vi "Drive GetSensors.vi"(1 "Drive Global Data In":T1) -> (0 "Drive Global Data Out":T1)   [LabVIEW 2013]
panel:
  in  "wheel diameteres":dbl
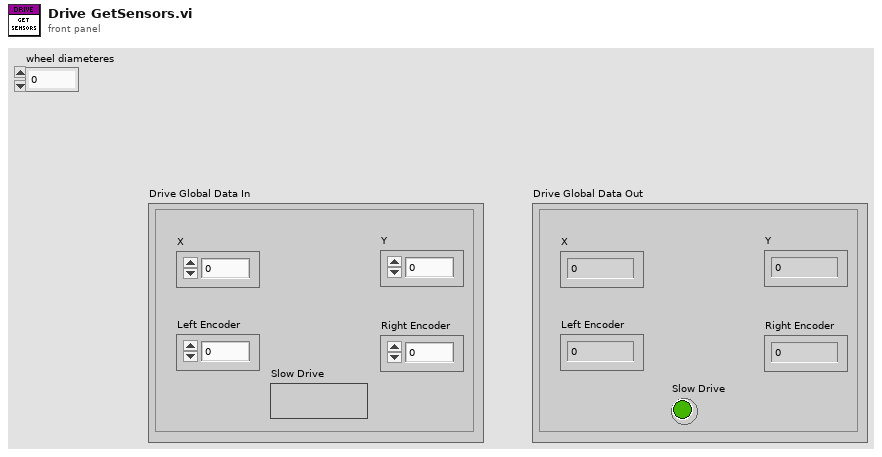
[diagram p1: front panel]
types:
  T1 = cluster{"Y":dbl, "X":dbl, "Left Encoder":dbl, "Right Encoder":dbl, "Slow Drive":bool}
  T2 = typedef "WPI_EncoderDevRef.ctl" = cluster{"DevStatus":errorcluster, "EncoderIndex":T3, "CounterIndex":T4, "DistancePerCount":dbl, "Decoding Type":T5}
  T3 = typedef "FPGA_EncoderIdx.ctl" = enum8{"Enc 0", "Enc 1", "Enc 2", "Enc 3", "Invalid"}
  T4 = typedef "FPGA_CounterCtrSystemIndex.ctl" = enum8{"Ctr 0", "Ctr 1", "Ctr 2", "Ctr 3", "Ctr 4", "Ctr 5", "Ctr 6", "Ctr 7", "Invalid"}
  T5 = typedef "WPI_EncoderType.ctl" = enum16{"1x", "2x", "4x"}
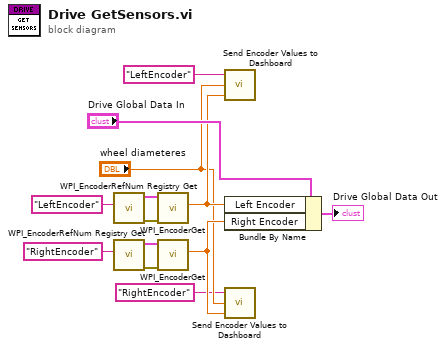
[diagram p0: block diagram]
diagram:
  n1 = call <vilib>:"WPI_EncoderRefNum Registry Get.vi"("refnum name"="LeftEncoder") -> ("error out"=w10:errorcluster, "EncoderDevRef"=w6:T2)  [unwired: 9 in]
  n2 = call <vilib>:"WPI_EncoderRefNum Registry Get.vi"("refnum name"="RightEncoder") -> ("error out"=w9:errorcluster, "EncoderDevRef"=w7:T2)  [unwired: 9 in]
  n3 = call <vilib>:"WPI_EncoderGet.vi"("error in (no error)"=w10, "EncoderDevRef"=w6) -> ("Distance"=w5:dbl)  [unwired: 4 in, 5 out]
  n4 = call <vilib>:"WPI_EncoderGet.vi"("error in (no error)"=w9, "EncoderDevRef"=w7) -> ("Distance"=w4:dbl)  [unwired: 4 in, 5 out]
  n5 = call "Send Encoder Values to Dashboard.vi"("Encoder Value"=w5, "wheel diameteres"="wheel diameteres", "Endcoder Name"="LeftEncoder" ("refnum name")) -> ()  [unwired: 1 in]
  n6 = Bundle By Name(cluster="Drive Global Data In", "Left Encoder"=w5, "Right Encoder"=w4) -> (→"Drive Global Data Out":T1)
  n7 = call "Send Encoder Values to Dashboard.vi"("Encoder Value"=w4, "wheel diameteres"="wheel diameteres", "Endcoder Name"="RightEncoder" ("refnum name")) -> ()  [unwired: 1 in]
